vi "column count.vi"(8 "error in (no error)":errorcluster, 11 "pStmt":u64) -> (0 "error out":errorcluster, 2 "#cols":i32, 3 "pStmt out":u64)   [LabVIEW 2020, in "sqlite3.lvlib"]
uses:
  sqlite3.lvlib
  bin/sqlite3_64.dll
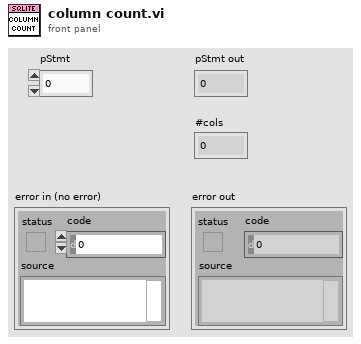
[diagram p1: front panel]
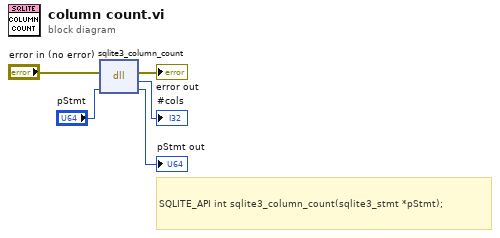
[diagram p0: block diagram]
diagram:
  # "SQLITE_API int sqlite3_column_count(sqlite3_stmt *pStmt);"
  n1 = dll-call lib="D:/Project/Labview-Projects/database-configuration/externals/sqlite3/Source/bin/sqlite3_*.*" fn="sqlite3_column_count"(error in="error in (no error)", "pStmt"="pStmt") -> (error out=→"error out":errorcluster, "return type"=→"#cols":i32, "pStmt"=→"pStmt out":u64)  [unwired: 2 in, 1 out]
